vi "3.vi"() -> ()   [LabVIEW 2020]
panel:
  out "Boolean":bool
  in  "Couple":string
  in  "String":string
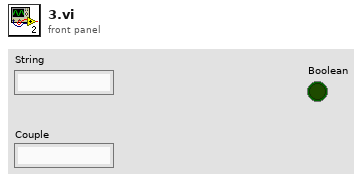
[diagram p1: front panel]
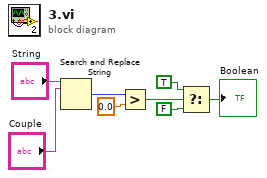
[diagram p0: block diagram]
diagram:
  n1 = Search and Replace String(input string="String", search string="Couple") -> (number of replacements=w5:i32)  [unwired: 6 in, 3 out]
  n2 = Greater?(x=w5, y=0.0) -> (0:w4:bool)
  n3 = Select(t=TRUE, s=w4, f=FALSE) -> (s? t:f=→"Boolean":bool)
